vi "setTriggerSequence.vi"(8 "error in (no error)":errorcluster, 10 "trigger_sequence":u16[](array[numeric]), 11 "Xcite in":refnum<class "Xcite.lvclass">) -> (0 "error out":errorcluster, 3 "Xcite out":refnum<class "Xcite.lvclass">)   [LabVIEW 2019, in "Xcite.lvclass"]
doc: "Sets the sequnce configuration of the X-Cite light source."
uses:
  Xcite.lvclass
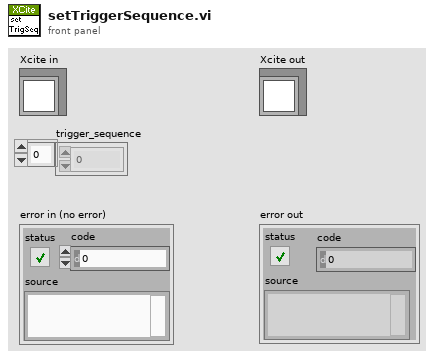
[diagram p1: front panel]
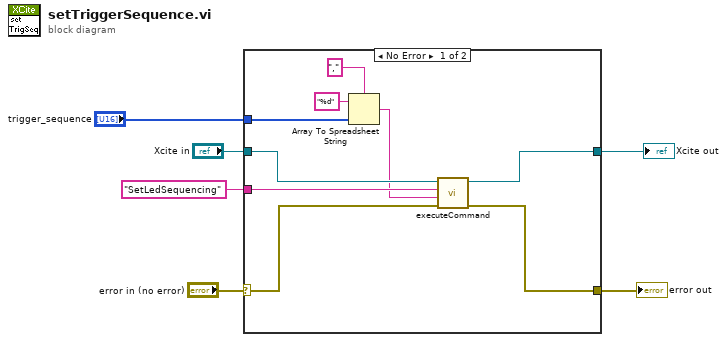
[diagram p0: block diagram]
diagram:
  n1 = case shown="No Error" "error in (no error)" {
    selector: "error in (no error)" -> [w11 w16]
    tunnel: "Xcite in" -> [w15 w17]
    tunnel: "SetLedSequencing" -> [w14 _]
    tunnel: [w13 w17] -> w4
    tunnel: [w12 w16] -> w3
    tunnel: "trigger_sequence" -> [w10 _]
    frame No Error {
      n2 = Array To Spreadsheet String(delimiter (Tab)=",", array=w10, 3:"%d" ("format string")) -> (spreadsheet string=w7:string)
      n3 = call "executeCommand.vi"("error in (no error)"=w11, "in_value"=w7, "cmd"=w14, "Xcite in"=w15) -> ("error out"=w12:errorcluster, "Xcite out"=w13:refnum<class "Xcite.lvclass">)  [unwired: 5 in, 1 out]
    }
    frame Error {
    }
  }
  "Xcite out" <- w4
  "error out" <- w3
